vi "log analysis_gps.vi"() -> ()   [LabVIEW 2019] (continued)
02000000,d426,15824;SOL_COMPUTED,L1_FLOAT,-1.000000000,81.985870361,-51.294281006,0.0,269.498687744,180.000000000,\"631T\",17,8,8,8,04,00,20,23*d2afce59\n\tsystem status\tnormal 2 27.900000 0 0\trobot status\t132.527983\t124.834671\t7.872000\t-0.704959\t-0.765344\t1.089934\t0.295000\t0.023000\n\t\n15:13:21.0\tlog_raw\tgps_raw\t#DUALANTENNAHEADINGA,USB3,0,49.5,FINESTEERING,2107,281619.000,02000000,d426,15824;SOL_COMPUTED,L1_FLOAT,-1.000000000,81.329711914,-49.084411621,0.0,261.078948975,180.000000000,\"631T\",18,8,8,8,04,00,20,23*0738c36d\n\tsystem status\tnormal 2 28.000000 0 0\trobot status\t132.671677\t124.829898\t7.873300\t-0.689398\t-0.745768\t1.834140\t0.257000\t0.090000\n\t\n15:13:21.5\tlog_raw\tgps_raw\t#DUALANTENNAHEADINGA,USB3,0,48.0,FINESTEERING,2107,281619.500,02000000,d426,15824;SOL_COMPUTED,NARROW_FLOAT,-1.000000000,83.428977966,-43.865173340,0.0,179.560241699,180.000000000,\"631T\",20,9,9,8,04,00,20,23*fb7ce078\n\tsystem status\tnormal 2 28.000000 0 0\trobot status\t132.812972\t124.826160\t7.871700\t-0.774766\t-0.698025\t2.416964\t0.284000\t0.023000\n\t\n15:13:22.0\tlog_raw\tgps_raw\t#DUALANTENNAHEADINGA,USB3,0,48.0,FINESTEERING,2107,281620.000,02000000,d426,15824;SOL_COMPUTED,NARROW_FLOAT,-1.000000000,83.177322388,-43.462402344,0.0,179.866409302,180.000000000,\"631T\",19,9,9,8,04,00,20,23*b83e1f1b\n\tsystem status\tnormal 2 28.100000 0 0\trobot status\t132.957208\t124.822783\t7.869900\t-0.755381\t-0.663432\t2.788208\t0.242000\t0.092000\n\t\n15:13:22.5\tlog_raw\tgps_raw\t#DUALANTENNAHEADINGA,USB3,0,44.5,FINESTEERING,2107,281620.500,02000000,d426,15824;SOL_COMPUTED,NARROW_FLOAT,-1.000000000,82.434860229,-53.334503174,0.0,202.841445923,166.629974365,\"631T\",18,8,8,8,04,00,20,23*e81d707d\n\tsystem status\tnormal 2 28.100000 0 0\trobot status\t133.098233\t124.820634\t7.869100\t-0.796184\t-0.528559\t3.164091\t0.414000\t-0.170000\n\t\n15:13:23.0\tlog_raw\tgps_raw\t#INSPVAXA,USB3,0,44.5,FINESTEERING,2107,281621.000,02000000,471d,15824;INS_ALIGNMENT_COMPLETE,INS_RTKFIXED,37.37125484776,126.72233928465,7.8682,22.3000,-0.0140,0.2874,-0.0021,-0.631288099,-0.470123008,86.597817260,0.4108,0.2750,0.5022,0.1095,0.0896,0.0746,0.1671,0.1681,5.1116,0f000001,0*0301d2b2\n\tsystem status\tnormal 2 28.100000 0 0\trobot status\t133.237761\t124.817911\t7.868200\t-0.631288\t-0.470123\t3.402183\t0.271000\t0.044000\n\t\n15:13:23.5\tlog_raw\tgps_raw\t#DUALANTENNAHEADINGA,USB3,0,47.5,FINESTEERING,2107,281621.500,02000000,d426,15824;SOL_COMPUTED,L1_FLOAT,-1.000000000,79.118186951,-47.831787109,0.0,285.028137207,180.000000000,\"631T\",21,8,8,8,04,00,20,23*eceb4aca\n\tsystem status\tnormal 2 28.100000 0 0\trobot status\t133.381909\t124.815038\t7.870000\t-0.413841\t-0.414727\t3.443892\t0.363000\t-0.086000\n\t\n15:13:24.0\tlog_raw\tgps_raw\t#DUALANTENNAHEADINGA,USB3,0,47.5,FINESTEERING,2107,281622.000,02000000,d426,15824;SOL_COMPUTED,L1_FLOAT,-1.000000000,79.215469360,-46.676361084,0.0,278.801727295,180.000000000,\"631T\",21,8,8,8,04,00,20,23*2f0de768\n\tsystem status\tnormal 2 28.200000 0 0\trobot status\t133.527421\t124.811541\t7.872000\t-0.238819\t-0.445818\t3.404348\t0.278000\t0.029000\n\t\n15:13:24.5\tlog_raw\tgps_raw\t#DUALANTENNAHEADINGA,USB3,0,50.0,FINESTEERING,2107,281622.500,02008000,d426,15824;SOL_COMPUTED,NARROW_FLOAT,-1.000000000,81.357048035,-52.184570313,0.0,156.938522339,171.573028564,\"631T\",22,8,8,8,04,00,20,23*a9a2e0bd\n\tsystem status\tnormal 2 28.200000 0 0\trobot status\t133.669990\t124.807065\t7.875800\t-0.115847\t-0.480549\t3.296523\t0.293000\t0.009000\n\t\n15:13:25.0\tlog_raw\tgps_raw\t#DUALANTENNAHEADINGA,USB3,0,50.0,FINESTEERING,2107,281623.000,02008000,d426,15824;SOL_COMPUTED,NARROW_FLOAT,-1.000000000,80.926651001,-50.941162109,0.0,157.099182129,180.000000000,\"631T\",22,8,8,8,04,00,20,23*29ef00a4\n\tsystem status\tnormal 2 28.200000 0 0\trobot status\t133.812784\t124.801470\t7.879500\t0.034583\t-0.554227\t3.198241\t0.295000\t-0.009000\n\t\n15:13:25.5\tlog_raw\tgps_raw\t#DUALANTENNAHEADINGA,USB3,0,47.0,FINESTEERING,2107,281623.500,02008000,d426,15824;SOL_COMPUTED,NARROW_FLOAT,-1.000000000,74.372909546,-36.647766113,0.0,211.228378296,180.000000000,\"631T\",21,9,9,8,04,00,20,23*0d510ff3\n\tsystem status\tnormal 2 28.200000 0 0\trobot status\t133.959682\t124.793507\t7.883200\t0.412890\t-0.814601\t3.103692\t0.299000\t-0.011000\n\t\n15:13:26.0\tlog_raw\tgps_raw\t#DUALANTENNAHEADINGA,USB3,0,47.0,FINESTEERING,2107,281624.000,02008000,d426,15824;SOL_COMPUTED,NARROW_FLOAT,-1.000000000,74.676368713,-33.559204102,0.0,205.690567017,180.000000000,\"631T\",20,9,9,8,04,00,20,23*f648ddb8\n\tsystem status\tnormal 2 28.200000 0 0\trobot status\t134.101094\t124.785415\t7.887300\t0.610602\t-0.952915\t3.005464\t0.297000\t-0.013000\n\t\n15:13:26.5\tlog_raw\tgps_raw\t#DUALANTENNAHEADINGA,USB3,0,47.5,FINESTEERING,2107,281624.500,02008000,d426,15824;SOL_COMPUTED,NARROW_FLOAT,-1.000000000,78.385162354,-52.385925293,0.0,193.963928223,180.000000000,\"631T\",19,8,8,8,04,00,20,23*14d467ea\n\tsystem status\tnormal 2 28.200000 0 0\trobot status\t134.242225\t124.778426\t7.889200\t0.752717\t-1.000787\t2.886940\t0.295000\t-0.016000\n\t\n15:13:27.0\tlog_raw\tgps_raw\t#DUALANTENNAHEADINGA,USB3,0,47.5,FINESTEERING,2107,281625.000,02008000,d426,15824;SOL_COMPUTED,NARROW_FLOAT,-1.000000000,78.697448730,-55.840881348,0.0,201.517425537,180.000000000,\"631T\",20,8,8,8,04,00,20,23*2125c3e9\n\tsystem status\tnormal 2 28.200000 0 0\trobot status\t134.384632\t124.770462\t7.890500\t0.886447\t-0.920314\t2.761621\t0.298000\t-0.007000\n\t\n15:13:27.5\tlog_raw\tgps_raw\t#DUALANTENNAHEADINGA,USB3,0,50.0,FINESTEERING,2107,281625.500,02008000,d426,15824;SOL_COMPUTED,NARROW_FLOAT,-1.000000000,76.255996704,-44.440551758,0.0,192.652679443,180.000000000,\"631T\",21,8,8,8,04,00,20,23*2ef6fdf0\n\tsystem status\tnormal 2 28.200000 0 0\trobot status\t134.527815\t124.762984\t7.891800\t1.028451\t-0.676309\t2.638165\t0.297000\t-0.013000\n\t\n15:13:28.0\tlog_raw\tgps_raw\t#DUALANTENNAHEADINGA,USB3,0,50.0,FINESTEERING,2107,281626.000,02008000,d426,15824;SOL_COMPUTED,NARROW_FLOAT,-1.000000000,76.051048279,-42.751831055,0.0,190.193801880,180.000000000,\"631T\",19,8,8,8,04,00,20,23*71df93c1\n\tsystem status\tnormal 2 28.200000 0 0\trobot status\t134.672251\t124.753527\t7.893800\t1.313181\t-0.400313\t2.489606\t0.294000\t-0.014000\n\t\n15:13:28.5\tlog_raw\tgps_raw\t\tsystem status\tnormal 2 28.200000 0 0\trobot status\t134.821411\t124.744984\t7.894300\t1.448971\t-0.286102\t2.371589\t0.296000\t-0.007000\n\t\n15:13:29.0\tlog_raw\tgps_raw\t#DUALANTENNAHEADINGA,USB3,0,49.0,FINESTEERING,2107,281627.000,02000000,d426,15824;SOL_COMPUTED,NARROW_FLOAT,-1.000000000,74.827011108,-47.434204102,0.0,215.584564209,180.000000000,\"631T\",20,6,6,6,04,00,20,03*11cc19a9\n\tsystem status\tnormal 2 28.200000 0 0\trobot status\t134.968968\t124.735417\t7.895300\t1.459946\t-0.353992\t2.207850\t0.302000\t-0.011000\n\t\n15:13:29.5\tlog_raw\tgps_raw\t#DUALANTENNAHEADINGA,USB3,0,50.0,FINESTEERING,2107,281627.500,02000000,d426,15824;SOL_COMPUTED,NARROW_FLOAT,-1.000000000,76.736885071,-60.461914063,0.0,257.944244385,180.000000000,\"631T\",20,6,6,6,04,00,20,03*64121f5a\n\tsystem status\tnormal 2 28.200000 0 0\trobot status\t135.110611\t124.726484\t7.897200\t1.391975\t-0.391573\t2.021625\t0.300000\t-0.012000\n\t\n15:13:30.0\tlog_raw\tgps_raw\t#DUALANTENNAHEADINGA,USB3,0,50.0,FINESTEERING,2107,281628.000,02000000,d426,15824;SOL_COMPUTED,NARROW_FLOAT,-1.000000000,76.336128235,-57.847045898,0.0,256.018859863,180.000000000,\"631T\",20,6,6,6,04,00,20,03*cae9a6c4\n\tsystem status\tnormal 2 28.200000 0 0\trobot status\t135.258314\t124.716625\t7.899300\t1.303987\t-0.581408\t1.863464\t0.296000\t-0.010000\n\t\n15:13:30.5\tlog_raw\tgps_raw\t#DUALANTENNAHEADINGA,USB3,0,49.0,FINESTEERING,2107,281628.500,02000000,d426,15824;SOL_COMPUTED,NARROW_FLOAT,-1.000000000,75.922164917,-51.811248779,0.0,196.475540161,180.000000000,\"631T\",21,6,6,6,04,00,20,03*71a30e30\n\tsystem status\tnormal 2 28.200000 0 0\trobot status\t135.405242\t124.709408\t7.900300\t1.225879\t-0.705011\t1.692036\t0.301000\t-0.006000\n\t\n15:13:31.0\tlog_raw\tgps_raw\t#DUALANTENNAHEADINGA,USB3,0,49.0,FINESTEERING,2107,281629.000,02000000,d426,15824;SOL_COMPUTED,NARROW_FLOAT,-1.000000000,75.688812256,-51.816131592,0.0,200.071166992,180.000000000,\"631T\",21,6,6,6,04,00,20,03*05442491\n\tsystem status\tnormal 2 28.200000 0 0\trobot status\t135.549471\t124.701412\t7.901000\t1.137564\t-0.721640\t1.522246\t0.302000\t-0.011000\n\t\n15:13:31.5\tlog_raw\tgps_raw\t#DUALANTENNAHEADINGA,USB3,0,47.0,FINESTEERING,2107,281629.500,02000000,d426,15824;SOL_COMPUTED,NARROW_FLOAT,-1.000000000,76.706954956,-45.822814941,0.0,158.336380005,180.000000000,\"631T\",21,7,7,6,04,00,20,03*a7b53285\n\tsystem status\tnormal 2 28.200000 0 0\trobot status\t135.689730\t124.694593\t7.901700\t1.081795\t-0.675095\t1.331584\t0.298000\t-0.003000\n\t\n15:13:32.0\tlog_raw\tgps_raw\t#DUALANTENNAHEADINGA,USB3,0,47.0,FINESTEERING,2107,281630.000,02000000,d426,15824;SOL_COMPUTED,NARROW_FLOAT,-1.000000000,76.392150879,-45.545715332,0.0,160.233947754,180.000000000,\"631T\",20,7,7,6,04,00,20,03*a337a603\n\tsystem status\tnormal 2 28.200000 0 0\trobot status\t135.832695\t124.687325\t7.902200\t0.907226\t-0.591803\t1.171661\t0.292000\t0.000000\n\t\n15:13:32.5\tlog_raw\tgps_raw\t#DUALANTENNAHEADINGA,USB3,0,50.0,FINESTEERING,2107,281630.500,02000000,d426,15824;SOL_COMPUTED,NARROW_FLOAT,-1.000000000,73.576385498,-34.237976074,0.0,224.892852783,180.000000000,\"631T\",20,7,7,6,04,00,20,03*509d4fa7\n\tsystem status\tnormal 2 28.200000 0 0\trobot status\t135.975938\t124.680414\t7.903900\t0.750666\t-0.654550\t1.015174\t0.302000\t-0.002000\n\t\n15:13:33.0\tlog_raw\tgps_raw\t#DUALANTENNAHEADINGA,USB3,0,50.0,FINESTEERING,2107,281631.000,02000000,d426,15824;SOL_COMPUTED,NARROW_FLOAT,-1.000000000,73.801551819,-34.781646729,0.0,227.056274414,180.000000000,\"631T\",20,7,7,6,04,00,20,03*62a89227\n\tsystem status\tnormal 2 28.200000 0 0\trobot status\t136.111228\t124.672284\t7.907100\t0.620165\t-0.528572\t0.833307\t0.298000\t0.000000\n\t\n15:13:33.5\tlog_raw\tgps_raw\t#DUALANTENNAHEADINGA,USB3,0,48.5,FINESTEERING,2107,281631.500,02000000,d426,15824;SOL_COMPUTED,NARROW_FLOAT,-1.000000000,72.331886292,-39.270935059,0.0,208.219329834,180.000000000,\"631T\",20,6,6,6,04,00,20,03*b4f25b02\n\tsystem status\tnormal 2 28.200000 0 0\trobot status\t136.251123\t124.665216\t7.908000\t0.625068\t-0.387180\t0.705750\t0.296000\t0.006000\n\t\n15:13:34.0\tlog_raw\tgps_raw\t#DUALANTENNAHEADINGA,USB3,0,48.5,FINESTEERING,2107,281632.000,02000000,d426,15824;SOL_COMPUTED,NARROW_FLOAT,-1.000000000,72.392997742,-44.277435303,0.0,216.308242798,180.000000000,\"631T\",20,6,6,6,04,00,20,03*f92d3de0\n\tsystem status\tnormal 2 28.200000 0 0\trobot status\t136.388999\t124.657518\t7.909100\t0.522944\t-0.320117\t0.535098\t0.295000\t-0.005000\n\t\n15:13:34.5\tlog_raw\tgps_raw\t#DUALANTENNAHEADINGA,USB3,0,50.5,FINESTEERING,2107,281632.500,02000000,d426,15824;SOL_COMPUTED,NARROW_FLOAT,-1.000000000,70.524742126,-43.222106934,0.0,187.663330078,180.000000000,\"631T\",20,6,6,6,04,00,20,03*23e53db0\n\tsystem status\tnormal 2 28.200000 0 0\trobot status\t136.527493\t124.649932\t7.910000\t0.480007\t-0.230660\t0.402714\t0.302000\t-0.002000\n\t\n15:13:35.0\tlog_raw\tgps_raw\t\tsystem status\tnormal 2 28.200000 0 0\trobot status\t136.664747\t124.641530\t7.912700\t0.383209\t-0.068987\t0.273789\t0.299000\t0.000000\n\t\n15:13:35.5\tlog_raw\tgps_raw\t\tsystem status\tnormal 2 28.200000 0 0\trobot status\t136.804079\t124.633410\t7.915200\t0.323321\t0.031538\t0.175839\t0.295000\t0.000000\n\t\n15:13:36.0\tlog_raw\tgps_raw\t\tsystem status\tnormal 2 28.200000 0 0\trobot status\t136.946767\t124.624659\t7.917300\t0.214120\t0.032979\t0.078057\t0.301000\t0.004000\n\t\n15:13:36.5\tlog_raw\tgps_raw\t#DUALANTENNAHEADINGA,USB3,0,49.5,FINESTEERING,2107,281634.500,02000000,d426,15824;SOL_COMPUTED,NARROW_FLOAT,-1.000000000,74.599754333,-34.968170166,0.0,186.703521729,180.000000000,\"631T\",21,8,8,8,04,00,20,33*c6f47f17\n\tsystem status\tnormal 2 28.200000 0 0\trobot status\t137.089583\t124.616962\t7.919700\t0.037424\t-0.007948\t-0.020745\t0.304000\t0.008000\n\t\n15:13:37.0\tlog_raw\tgps_raw\t#DUALANTENNAHEADINGA,USB3,0,49.5,FINESTEERING,2107,281635.000,02000000,d426,15824;SOL_COMPUTED,NARROW_FLOAT,-1.000000000,74.584259033,-34.924865723,0.0,186.240829468,180.000000000,\"631T\",21,8,8,8,04,00,20,33*9c697b75\n\tsystem status\tnormal 2 28.200000 0 0\trobot status\t137.230387\t124.607716\t7.921700\t-0.027327\t-0.162985\t-0.124730\t0.299000\t0.008000\n\t\n15:13:37.5\tlog_raw\tgps_raw\t#DUALANTENNAHEADINGA,USB3,0,46.5,FINESTEERING,2107,281635.500,02000000,d426,15824;SOL_COMPUTED,NARROW_FLOAT,-1.000000000,67.143241882,-41.090057373,0.0,270.678344727,180.000000000,\"631T\",21,8,8,8,04,00,20,23*92e43030\n\tsystem status\tnormal 2 28.200000 0 0\trobot status\t137.372263\t124.599397\t7.922900\t-0.076547\t-0.321066\t-0.217362\t0.301000\t0.007000\n\t\n15:13:38.0\tlog_raw\tgps_raw\t#INSPVAXA,USB3,0,46.5,FINESTEERING,2107,281636.050,02000000,471d,15824;INS_ALIGNMENT_COMPLETE,INS_RTKFIXED,37.37125277821,126.72238773089,7.9249,22.3000,-0.0472,0.2751,0.0261,0.033461112,-0.337994912,90.276833598,0.4107,0.2743,0.5040,0.1102,0.0902,0.0747,0.1666,0.1669,5.1095,0f000001,0*fb0d7dd5\n\tsystem status\tnormal 2 28.200000 0 0\trobot status\t137.529050\t124.588153\t7.924900\t0.033461\t-0.337995\t-0.276834\t0.298000\t0.005000\n\t\n15:13:38.5\tlog_raw\tgps_raw\t#INSPVAXA,USB3,0,49.0,FINESTEERING,2107,281636.550,02000000,471d,15824;INS_ALIGNMENT_COMPLETE,INS_RTKFIXED,37.37125270683,126.72238933988,7.9258,22.3000,-0.0404,0.2826,0.0202,-0.092396581,-0.312496368,90.344441421,0.4107,0.2743,0.5040,0.1102,0.0902,0.0747,0.1666,0.1669,5.1095,0f000001,0*2ea03c91\n\tsystem status\tnormal 2 28.200000 0 0\trobot status\t137.671572\t124.580228\t7.925800\t-0.092397\t-0.312496\t-0.344441\t0.304000\t0.006000\n\t\n15:13:39.0\tlog_raw\tgps_raw\t\tsystem status\tnormal 2 28.200000 0 0\trobot status\t137.796732\t124.571946\t7.926200\t-0.126269\t-0.143738\t-0.384547\t0.296000\t0.008000\n\t\n15:13:39.5\tlog_raw\tgps_raw\t\tsystem status\tnormal 2 28.200000 0 0\trobot status\t137.940609\t124.562478\t7.926700\t-0.091947\t-0.054945\t-0.381561\t0.244000\t0.066000\n\t\n15:13:40.0\tlog_raw\tgps_raw\t#DUALANTENNAHEADINGA,USB3,0,45.5,FINESTEERING,2107,281638.000,02000000,d426,15824;SOL_COMPUTED,L1_FLOAT,-1.000000000,68.590065002,-38.051055908,0.0,183.932281494,180.000000000,\"631T\",19,6,6,6,04,00,20,03*7caf4eb9\n\tsystem status\tnormal 2 28.200000 0 0\trobot status\t138.081185\t124.552915\t7.928500\t-0.095749\t-0.090492\t-0.295128\t0.301000\t0.006000\n\t\n15:13:40.5\tlog_raw\tgps_raw\t#DUALANTENNAHEADINGA,USB3,0,46.5,FINESTEERING,2107,281638.500,02000000,d426,15824;SOL_COMPUTED,NARROW_FLOAT,-1.000000000,65.883399963,-37.877685547,0.0,260.404785156,180.000000000,\"631T\",19,6,6,6,04,00,20,03*2dc9451b\n\tsystem status\tnormal 2 28.200000 0 0\trobot status\t138.222022\t124.543481\t7.929100\t-0.131894\t-0.163924\t-0.209489\t0.369000\t-0.101000\n\t\n15:13:41.0\tlog_raw\tgps_raw\t#DUALANTENNAHEADINGA,USB3,0,46.5,FINESTEERING,2107,281639.000,02000000,d426,15824;SOL_COMPUTED,NARROW_FLOAT,-1.000000000,66.000267029,-38.685607910,0.0,260.610321045,180.000000000,\"631T\",20,6,6,6,04,00,20,03*4d0efe6f\n\tsystem status\tnormal 2 28.200000 0 0\trobot status\t138.363859\t124.533398\t7.929800\t-0.101029\t-0.169552\t-0.100452\t0.253000\t0.068000\n\t\n15:13:41.5\tlog_raw\tgps_raw\t#DUALANTENNAHEADINGA,USB3,0,48.5,FINESTEERING,2107,281639.500,02000000,d426,15824;SOL_COMPUTED,L1_FLOAT,-1.000000000,75.249496460,-42.510375977,0.0,208.045684814,180.000000000,\"631T\",21,6,6,6,04,00,20,03*5f68b654\n\tsystem status\tnormal 2 28.100000 0 0\trobot status\t138.507917\t124.525404\t7.930000\t-0.080780\t-0.161525\t0.054370\t0.379000\t-0.118000\n\t\n15:13:42.0\tlog_raw\tgps_raw\t#INSPVAXA,USB3,0,48.5,FINESTEERING,2107,281640.050,02000000,471d,15824;INS_ALIGNMENT_COMPLETE,INS_RTKFIXED,37.37125214763,126.72240056337,7.9297,22.3000,-0.0135,0.2579,0.0068,-0.286062471,-0.323666659,89.847152280,0.4125,0.2764,0.5060,0.1103,0.0900,0.0751,0.1666,0.1668,5.0988,0f000001,0*ba23ac07\n\tsystem status\tnormal 2 28.100000 0 0\trobot status\t138.665730\t124.518149\t7.929700\t-0.286062\t-0.323667\t0.152848\t0.293000\t0.019000\n\t\n15:13:42.5\tlog_raw\tgps_raw\t#INSPVAXA,USB3,0,48.0,FINESTEERING,2107,281640.550,02000000,471d,15824;INS_ALIGNMENT_COMPLETE,INS_RTKFIXED,37.37125209177,126.72240219164,7.9302,22.3000,-0.0088,0.2910,0.0070,-0.402825577,-0.342049421,89.793656004,0.4125,0.2764,0.5060,0.1103,0.0900,0.0751,0.1666,0.1668,5.0988,0f000001,0*83e377ec\n\tsystem status\tnormal 2 28.100000 0 0\trobot status\t138.809960\t124.511947\t7.930200\t-0.402826\t-0.342049\t0.206344\t0.297000\t0.007000\n\t\n15:13:43.0\tlog_raw\tgps_raw\t\tsystem status\tnormal 2 28.100000 0 0\trobot status\t138.938093\t124.505250\t7.930200\t-0.365984\t-0.316955\t0.417263\t0.357000\t-0.091000\n\t\n15:13:43.5\tlog_raw\tgps_raw\t\tsystem status\tnormal 2 28.100000 0 0\trobot status\t139.083168\t124.498292\t7.930000\t-0.534292\t-0.438853\t0.507811\t0.211000\t0.110000\n\t\n15:13:44.0\tlog_raw\tgps_raw\t\tsystem status\tnormal 2 28.100000 0 0\trobot status\t139.226269\t124.491404\t7.929600\t-0.722782\t-0.398658\t0.533081\t0.406000\t-0.162000\n\t\n15:13:44.5\tlog_raw\tgps_raw\t\tsystem status\tnormal 2 28.200000 0 0\trobot status\t139.369835\t124.484513\t7.927700\t-0.695260\t-0.251085\t0.563271\t0.261000\t0.043000\n\t\n15:13:45.0\tlog_raw\tgps_raw\t#INSPVAXA,USB3,0,49.5,FINESTEERING,2107,281643.050,02000000,471d,15824;INS_ALIGNMENT_COMPLETE,INS_RTKFIXED,37.37125177239,126.72241029930,7.9253,22.3000,-0.0184,0.2626,0.0057,-0.672263501,-0.094085877,89.482974840,0.4115,0.2769,0.5079,0.1098,0.0898,0.0750,0.1665,0.1668,5.0987,0f000001,0*08f45476\n\tsystem status\tnormal 2 28.100000 0 0\trobot status\t139.528123\t124.476489\t7.925300\t-0.672264\t-0.094086\t0.517025\t0.352000\t-0.107000\n\t\n15:13:45.5\tlog_raw\tgps_raw\t\tsystem status\tnormal 2 28.200000 0 0\trobot status\t139.657963\t124.469457\t7.924200\t-0.620368\t-0.040100\t0.509446\t0.290000\t0.006000\n\t\n15:13:46.0\tlog_raw\tgps_raw\t#INSPVAXA,USB3,0,45.0,FINESTEERING,2107,281644.050,02000000,471d,15824;INS_ALIGNMENT_COMPLETE,INS_RTKFIXED,37.37125163862,126.72241353138,7.9238,22.3000,-0.0195,0.2934,0.0047,-0.764058138,0.046945351,89.556014373,0.4117,0.2771,0.5083,0.1098,0.0898,0.0750,0.1665,0.1667,5.0999,0f000001,0*ca60484a\n\tsystem status\tnormal 2 28.200000 0 0\trobot status\t139.814415\t124.461638\t7.923800\t-0.764058\t0.046945\t0.443986\t0.313000\t-0.019000\n\t\n15:13:46.5\tlog_raw\tgps_raw\t#INSPVAXA,USB3,0,49.0,FINESTEERING,2107,281644.550,02000000,471d,15824;INS_ALIGNMENT_COMPLETE,INS_RTKFIXED,37.37125159291,126.72241516710,7.9252,22.3000,-0.0125,0.2656,0.0050,-0.825704601,0.105733929,89.608837523,0.4117,0.2771,0.5083,0.1098,0.0898,0.0750,0.1665,0.1667,5.0999,0f000001,0*afd891ca\n\tsystem status\tnormal 2 28.200000 0 0\trobot status\t139.959304\t124.456563\t7.925200\t-0.825705\t0.105734\t0.391162\t0.286000\t-0.009000\n\t\n15:13:47.0\tlog_raw\tgps_raw\t#INSPVAXA,USB3,0,49.0,FINESTEERING,2107,281645.050,02000000,471d,15824;INS_ALIGNMENT_COMPLETE,INS_RTKFIXED,37.37125153841,126.72241684941,7.9264,22.3000,-0.0138,0.2766,0.0005,-0.782015483,0.115845462,89.701566718,0.4112,0.2772,0.5084,0.1097,0.0898,0.0750,0.1665,0.1667,5.1015,0f000001,0*e301f266\n\tsystem status\tnormal 2 28.200000 0 0\trobot status\t140.108321\t124.450511\t7.926400\t-0.782015\t0.115845\t0.298433\t0.294000\t-0.003000\n\t\n15:13:47.5\tlog_raw\tgps_raw\t\tsystem status\tnormal 2 28.200000 0 0\trobot status\t140.237450\t124.444010\t7.925800\t-0.680854\t-0.008764\t0.272391\t0.302000\t-0.013000\n\t\n15:13:48.0\tlog_raw\tgps_raw\t#INSPVAXA,USB3,0,51.0,FINESTEERING,2107,281646.050,02000000,471d,15824;INS_ALIGNMENT_COMPLETE,INS_RTKFIXED,37.37125141044,126.72242010916,7.9241,22.3000,-0.0145,0.2894,0.0046,-0.683948152,-0.106427214,89.829684662,0.4110,0.2773,0.5083,0.1096,0.0899,0.0750,0.1665,0.1667,5.1032,0f000001,0*7e3f8e98\n\tsystem status\tnormal 2 28.200000 0 0\trobot status\t140.397064\t124.436304\t7.924100\t-0.683948\t-0.106427\t0.170315\t0.295000\t-0.013000\n\t\n15:13:48.5\tlog_raw\tgps_raw\t\tsystem status\tnormal 2 28.200000 0 0\trobot status\t140.529109\t124.428553\t7.922100\t-0.559415\t-0.144844\t0.061968\t0.288000\t-0.017000\n\t\n15:13:49.0\tlog_raw\tgps_raw\t\tsystem status\tnormal 2 28.200000 0 0\trobot status\t140.670749\t124.420683\t7.920600\t-0.646021\t-0.153969\t-0.024187\t0.298000\t-0.013000\n\t\n15:13:49.5\tlog_raw\tgps_raw\t\tsystem status\tnormal 2 28.200000 0 0\trobot status\t140.810969\t124.412523\t7.920300\t-0.671934\t0.006720\t-0.060655\t0.301000\t-0.013000\n\t\n15:13:50.0\tlog_raw\tgps_raw\t\tsystem status\tnormal 2 28.200000 0 0\trobot status\t140.956641\t124.403565\t7.920000\t-0.694143\t0.279069\t-0.163248\t0.292000\t-0.017000\n\t\n15:13:50.5\tlog_raw\tgps_raw\t#INSPVAXA,USB3,0,50.5,FINESTEERING,2107,281648.550,02000000,471d,15824;INS_ALIGNMENT_COMPLETE,INS_RTKFIXED,37.37125104211,126.72242819820,7.9192,22.3000,-0.0057,0.2779,0.0043,-0.865746254,0.658403910,90.332036751,0.4101,0.2775,0.5080,0.1095,0.0899,0.0749,0.1664,0.1667,5.1060,0f000001,0*c1bd000c\n\tsystem status\tnormal 2 28.200000 0 0\trobot status\t141.113578\t124.395413\t7.919200\t-0.865746\t0.658404\t-0.332037\t0.298000\t-0.011000\n\t\n15:13:51.0\tlog_raw\tgps_raw\t#INSPVAXA,USB3,0,47.0,FINESTEERING,2107,281649.050,02000000,471d,15824;INS_ALIGNMENT_COMPLETE,INS_RTKFIXED,37.37125095950,126.72242975720,7.9195,22.3000,-0.0170,0.2957,0.0033,-0.943502690,0.808287959,90.436788993,0.4102,0.2776,0.5078,0.1095,0.0899,0.0749,0.1664,0.1667,5.1072,0f000001,0*5974bd17\n\tsystem status\tnormal 2 28.200000 0 0\trobot status\t141.251672\t124.386242\t7.919500\t-0.943503\t0.808288\t-0.436789\t0.297000\t-0.013000\n\t\n15:13:51.5\tlog_raw\tgps_raw\t#INSPVAXA,USB3,0,47.0,FINESTEERING,2107,281649.550,02000000,471d,15824;INS_ALIGNMENT_COMPLETE,INS_RTKFIXED,37.37125085766,126.72243133912,7.9203,22.3000,-0.0165,0.2929,0.0110,-0.815482674,0.895195605,90.550000781,0.4102,0.2776,0.5078,0.1095,0.0899,0.0749,0.1664,0.1667,5.1072,0f000001,0*975e6869\n\tsystem status\tnormal 2 28.200000 0 0\trobot status\t141.391796\t124.374937\t7.920300\t-0.815483\t0.895196\t-0.550001\t0.294000\t-0.017000\n\t\n15:13:52.0\tlog_raw\tgps_raw\t#INSPVAXA,USB3,0,47.0,FINESTEERING,2107,281650.050,02000000,471d,15824;INS_ALIGNMENT_COMPLETE,INS_RTKFIXED,37.37125074410,126.72243299345,7.9208,22.3000,-0.0194,0.2944,0.0151,-0.654661826,0.805584356,90.730688305,0.4111,0.2776,0.5078,0.1096,0.0901,0.0749,0.1664,0.1667,5.1084,0f000001,0*7ee54a6b\n\tsystem status\tnormal 2 28.200000 0 0\trobot status\t141.538333\t124.362331\t7.920800\t-0.654662\t0.805584\t-0.730688\t0.292000\t-0.013000\n\t\n15:13:52.5\tlog_raw\tgps_raw\t#INSPVAXA,USB3,0,49.5,FINESTEERING,2107,281650.550,02000000,471d,15824;INS_ALIGNMENT_COMPLETE,INS_RTKFIXED,37.37125062801,126.72243464345,7.9218,22.3000,-0.0206,0.2968,0.0101,-0.581641852,0.404768185,90.963959440,0.4111,0.2776,0.5078,0.1096,0.0901,0.0749,0.1664,0.1667,5.1084,0f000001,0*f2a4c14e\n\tsystem status\tnormal 2 28.200000 0 0\trobot status\t141.684488\t124.349444\t7.921800\t-0.581642\t0.404768\t-0.963959\t0.299000\t-0.009000\n\t\n15:13:53.0\tlog_raw\tgps_raw\t#INSPVAXA,USB3,0,49.5,FINESTEERING,2107,281651.050,02000000,471d,15824;INS_ALIGNMENT_COMPLETE,INS_RTKFIXED,37.37125051285,126.72243625014,7.9235,22.3000,-0.0268,0.3045,0.0175,-0.662592503,0.202583400,91.123013334,0.4115,0.2778,0.5076,0.1098,0.0901,0.0749,0.1663,0.1667,5.1090,0f000001,0*216f234f\n\tsystem status\tnormal 2 28.200000 0 0\trobot status\t141.826806\t124.336661\t7.923500\t-0.662593\t0.202583\t-1.123013\t0.302000\t-0.010000\n\t\n15:13:53.5\tlog_raw\tgps_raw\t\tsystem status\tnormal 2 28.200000 0 0\trobot status\t141.956980\t124.325325\t7.923600\t-0.638179\t0.078223\t-1.263436\t0.295000\t-0.003000\n\t\n15:13:54.0\tlog_raw\tgps_raw\t#INSPVAXA,USB3,0,45.5,FINESTEERING,2107,281652.050,02000000,471d,15824;INS_ALIGNMENT_COMPLETE,INS_RTKFIXED,37.37125028624,126.72243951930,7.9245,22.3000,-0.0369,0.2898,0.0166,-0.721183306,0.056680654,91.387520198,0.4416,0.2813,0.5208,0.1150,0.0908,0.0760,0.1664,0.1673,5.1091,0f000001,0*25228c2c\n\tsystem status\tnormal 2 28.200000 0 0\trobot status\t142.116382\t124.311506\t7.924500\t-0.721183\t0.056681\t-1.387520\t0.304000\t-0.005000\n\t\n15:13:54.5\tlog_raw\tgps_raw\t\tsystem status\tnormal 2 28.200000 0 0\trobot status\t142.244213\t124.299152\t7.925200\t-0.610039\t0.089492\t-1.534593\t0.296000\t-0.010000\n\t\n15:13:55.0\tlog_raw\tgps_raw\t#INSPVAXA,USB3,0,47.5,FINESTEERING,2107,281653.050,02000000,471d,15824;INS_ALIGNMENT_COMPLETE,INS_RTKFIXED,37.37125003154,126.72244272682,7.9262,22.3000,-0.0470,0.2934,0.0145,-0.464349418,0.202545011,91.639204054,0.4699,0.2842,0.5361,0.1187,0.0913,0.0769,0.1664,0.1677,5.1090,0f000001,0*2b109b71\n\tsystem status\tnormal 2 28.200000 0 0\trobot status\t142.400499\t124.283233\t7.926200\t-0.464349\t0.202545\t-1.639204\t0.302000\t0.000000\n\t\n15:13:55.5\tlog_raw\tgps_raw\t#INSPVAXA,USB3,0,47.5,FINESTEERING,2107,281653.550,02000000,471d,15824;INS_ALIGNMENT_COMPLETE,INS_RTKFIXED,37.37124990486,126.72244436292,7.9283,22.3000,-0.0470,0.2912,0.0231,-0.374405811,0.178417245,91.756627389,0.4699,0.2842,0.5361,0.1187,0.0913,0.0769,0.1664,0.1677,5.1090,0f000001,0*1daf5624\n\tsystem status\tnormal 2 28.200000 0 0\trobot status\t142.545422\t124.269171\t7.928300\t-0.374406\t0.178417\t-1.756627\t0.304000\t-0.001000\n\t\n15:13:56.0\tlog_raw\tgps_raw\t#INSPVAXA,USB3,0,47.5,FINESTEERING,2107,281654.050,02000000,471d,15824;INS_ALIGNMENT_COMPLETE,INS_RTKFIXED,37.37124978665,126.72244599017,7.9303,22.3000,-0.0443,0.2911,0.0221,-0.533917833,0.012272263,91.868776619,0.4905,0.2861,0.5500,0.1206,0.0913,0.0777,0.1663,0.1679,5.1083,0f000001,0*b5797700\n\tsystem status\tnormal 2 28.200000 0 0\trobot status\t142.689562\t124.256049\t7.930300\t-0.533918\t0.012272\t-1.868777\t0.303000\t0.003000\n\t\n15:13:56.5\tlog_raw\tgps_raw\t#INSPVAXA,USB3,0,50.0,FINESTEERING,2107,281654.550,02000000,471d,15824;INS_ALIGNMENT_COMPLETE,INS_RTKFIXED,37.37124968143,126.72244761542,7.9319,22.3000,-0.0412,0.3115,0.0211,-0.670904223,-0.153080533,91.963880825,0.4905,0.2861,0.5500,0.1206,0.0913,0.0777,0.1663,0.1679,5.1083,0f000001,0*92b26d05\n\tsystem status\tnormal 2 28.200000 0 0\trobot status\t142.833524\t124.244369\t7.931900\t-0.670904\t-0.153081\t-1.963881\t0.302000\t0.006000\n\t\n15:13:57.0\tlog_raw\tgps_raw\t#INSPVAXA,USB3,0,50.0,FINESTEERING,2107,281655.050,02000000,471d,15824;INS_ALIGNMENT_COMPLETE,INS_RTKFIXED,37.37124956365,126.72244929570,7.9335,22.3000,-0.0287,0.2866,0.0163,-0.633101230,-0.384686660,92.084311938,0.4910,0.2854,0.5548,0.1194,0.0909,0.0776,0.1663,0.1676,5.1075,0f000001,0*34863e77\n\tsystem status\tnormal 2 28.200000 0 0\trobot status\t142.982360\t124.231295\t7.933500\t-0.633101\t-0.384687\t-2.084312\t0.297000\t0.000000\n\t\n15:13:57.5\tlog_raw\tgps_raw\t#INSPVAXA,USB3,0,45.0,FINESTEERING,2107,281655.550,02000000,471d,15824;INS_ALIGNMENT_COMPLETE,INS_RTKFIXED,37.37124945994,126.72245094764,7.9362,22.3000,-0.0311,0.2897,0.0132,-0.611375277,-0.501090520,92.141784733,0.4910,0.2854,0.5548,0.1194,0.0909,0.0776,0.1663,0.1676,5.1075,0f000001,0*d10d29d1\n\tsystem status\tnormal 2 28.200000 0 0\trobot status\t143.128686\t124.219782\t7.936200\t-0.611375\t-0.501091\t-2.141785\t0.299000\t0.006000\n\t\n15:13:58.0\tlog_raw\tgps_raw\t#INSPVAXA,USB3,0,45.0,FINESTEERING,2107,281656.050,02000000,471d,15824;INS_ALIGNMENT_COMPLETE,INS_RTKFIXED,37.37124935153,126.72245256975,7.9391,22.3000,-0.0386,0.2989,0.0132,-0.570389168,-0.459677112,92.213933334,0.4880,0.2845,0.5571,0.1182,0.0907,0.0775,0.1662,0.1674,5.1068,0f000001,0*a2bfb50c\n\tsystem status\tnormal 2 28.200000 0 0\trobot status\t143.272370\t124.207748\t7.939100\t-0.570389\t-0.459677\t-2.213933\t0.302000\t0.005000\n\t\n15:13:58.5\tlog_raw\tgps_raw\t\tsystem status\tnormal 2 28.200000 0 0\trobot status\t143.415453\t124.194029\t7.938500\t-0.577962\t-0.370357\t-2.256851\t0.300000\t0.004000\n\t\n15:13:59.0\tlog_raw\tgps_raw\t#INSPVAXA,USB3,0,48.5,FINESTEERING,2107,281657.050,02000000,471d,15824;INS_ALIGNMENT_COMPLETE,INS_RTKFIXED,37.37124909812,126.72245582569,7.9380,22.3000,-0.0275,0.2897,0.0035,-0.469663173,-0.125718508,92.311505672,0.4756,0.2829,0.5533,0.1158,0.0905,0.0770,0.1661,0.1672,5.1057,0f000001,0*07acf302\n\tsystem status\tnormal 2 28.200000 0 0\trobot status\t143.560776\t124.179618\t7.938000\t-0.469663\t-0.125719\t-2.311506\t0.300000\t0.006000\n\t\n15:13:59.5\tlog_raw\tgps_raw\t#INSPVAXA,USB3,0,45.5,FINESTEERING,2107,281657.550,02000000,471d,15824;INS_ALIGNMENT_COMPLETE,INS_RTKFIXED,37.37124898406,126.72245743531,7.9384,22.3000,-0.0303,0.2838,-0.0006,-0.590912103,0.021707043,92.352601821,0.4756,0.2829,0.5533,0.1158,0.0905,0.0770,0.1661,0.1672,5.1057,0f000001,0*08773687\n\tsystem status\tnormal 2 28.200000 0 0\trobot status\t143.703353\t124.166957\t7.938400\t-0.590912\t0.021707\t-2.352602\t0.283000\t0.026000\n\t\n15:14:00.0\tlog_raw\tgps_raw\t#INSPVAXA,USB3,0,45.5,FINESTEERING,2107,281658.050,02000000,471d,15824;INS_ALIGNMENT_COMPLETE,INS_RTKFIXED,37.37124887128,126.72245908204,7.9396,22.3000,-0.0216,0.3115,-0.0012,-0.683943291,-0.073848905,92.385513763,0.4705,0.2822,0.5519,0.1155,0.0906,0.0768,0.1661,0.1672,5.1055,0f000001,0*f6b19920\n\tsystem status\tnormal 2 28.200000 0 0\trobot status\t143.849218\t124.154437\t7.939600\t-0.683943\t-0.073849\t-2.385514\t0.313000\t-0.008000\n\t\n15:14:00.5\tlog_raw\tgps_raw\t#INSPVAXA,USB3,0,47.0,FINESTEERING,2107,281658.550,02000000,471d,15824;INS_ALIGNMENT_COMPLETE,INS_RTKFIXED,37.37124877139,126.72246069396,7.9391,22.3000,-0.0206,0.3045,-0.0060,-0.740293612,-0.175653816,92.281973521,0.4705,0.2822,0.5519,0.1155,0.0906,0.0768,0.1661,0.1672,5.1055,0f000001,0*bcff9c67\n\tsystem status\tnormal 2 28.100000 0 0\trobot status\t143.991999\t124.143349\t7.939100\t-0.740294\t-0.175654\t-2.281974\t0.362000\t-0.092000\n\t\n15:14:01.0\tlog_raw\tgps_raw\t#INSPVAXA,USB3,0,47.0,FINESTEERING,2107,281659.050,02000000,471d,15824;INS_ALIGNMENT_COMPLETE,INS_RTKFIXED,37.37124867854,126.72246232189,7.9387,22.3000,-0.0180,0.2907,0.0091,-0.761412694,-0.318240084,92.179006494,0.4753,0.2827,0.5554,0.1164,0.0908,0.0769,0.1661,0.1674,5.1056,0f000001,0*0b8ce59e\n\tsystem status\tnormal 2 28.200000 0 0\trobot status\t144.136199\t124.133041\t7.938700\t-0.761413\t-0.318240\t-2.179006\t0.275000\t0.038000\n\t\n15:14:01.5\tlog_raw\tgps_raw\t\tsystem status\tnormal 2 28.100000 0 0\trobot status\t144.281252\t124.120874\t7.938900\t-0.713124\t-0.523427\t-2.080293\t0.279000\t0.033000\n\t\n15:14:02.0\tlog_raw\tgps_raw\t#INSPVAXA,USB3,0,48.0,FINESTEERING,2107,281660.050,02000000,471d,15824;INS_ALIGNMENT_COMPLETE,INS_RTKFIXED,37.37124847032,126.72246556404,7.9397,22.3000,-0.0209,0.3095,-0.0013,-0.677978130,-0.485395170,91.982371596,0.4840,0.2835,0.5609,0.1180,0.0910,0.0772,0.1661,0.1676,5.1059,0f000001,0*3e0b93c3\n\tsystem status\tnormal 2 28.100000 0 0\trobot status\t144.423383\t124.109927\t7.939700\t-0.677978\t-0.485395\t-1.982372\t0.291000\t0.029000\n\t\n15:14:02.5\tlog_raw\tgps_raw\t#INSPVAXA,USB3,0,49.0,FINESTEERING,2107,281660.550,02000000,471d,15824;INS_ALIGNMENT_COMPLETE,INS_RTKFIXED,37.37124837512,126.72246716631,7.9375,22.3000,-0.0227,0.2996,0.0028,-0.584311559,-0.386112040,91.866898679,0.4840,0.2835,0.5609,0.1180,0.0910,0.0772,0.1661,0.1676,5.1059,0f000001,0*45e2577e\n\tsystem status\tnormal 2 28.100000 0 0\trobot status\t144.565309\t124.099359\t7.937500\t-0.584312\t-0.386112\t-1.866899\t0.292000\t0.024000\n\t\n15:14:03.0\tlog_raw\tgps_raw\t#INSPVAXA,USB3,0,48.0,FINESTEERING,2107,281661.050,02000000,471d,15824;INS_ALIGNMENT_COMPLETE,INS_RTKFIXED,37.37124829104,126.72246876695,7.9348,22.3000,-0.0195,0.3013,0.0019,-0.605545922,-0.315098575,91.766604977,0.4893,0.2839,0.5649,0.1187,0.0910,0.0774,0.1661,0.1677,5.1061,0f000001,0*33d9cb01\n\tsystem status\tnormal 2 28.100000 0 0\trobot status\t144.707091\t124.090025\t7.934800\t-0.605546\t-0.315099\t-1.766605\t0.290000\t0.021000\n\t\n15:14:03.5\tlog_raw\tgps_raw\t\tsystem status\tnormal 2 28.100000 0 0\trobot status\t144.850142\t124.079476\t7.935200\t-0.604211\t-0.237981\t-1.678856\t0.302000\t0.007000\n\t\n15:14:04.0\tlog_raw\tgps_raw\t#INSPVAXA,USB3,0,48.0,FINESTEERING,2107,281662.050,02000000,471d,15824;INS_ALIGNMENT_COMPLETE,INS_RTKFIXED,37.37124811177,126.72247195093,7.9364,22.3000,-0.0115,0.2979,0.0095,-0.572003488,-0.073343292,91.548333593,0.4907,0.2839,0.5665,0.1189,0.0910,0.0775,0.1660,0.1678,5.1065,0f000001,0*28865f95\n\tsystem status\tnormal 2 28.100000 0 0\trobot status\t144.989123\t124.070124\t7.936400\t-0.572003\t-0.073343\t-1.548334\t0.295000\t0.007000\n\t\n15:14:04.5\tlog_raw\tgps_raw\t#INSPVAXA,USB3,0,49.5,FINESTEERING,2107,281662.550,02000000,471d,15824;INS_ALIGNMENT_COMPLETE,INS_RTKFIXED,37.37124803275,126.72247354020,7.9355,22.3000,-0.0061,0.2831,0.0061,-0.496782272,0.001131440,91.456585867,0.4907,0.2839,0.5665,0.1189,0.0910,0.0775,0.1660,0.1678,5.1065,0f000001,0*47f56ed7\n\tsystem status\tnormal 2 28.100000 0 0\trobot status\t145.129898\t124.061351\t7.935500\t-0.496782\t0.001131\t-1.456586\t0.276000\t0.026000\n\t\n15:14:05.0\tlog_raw\tgps_raw\t#INSPVAXA,USB3,0,49.5,FINESTEERING,2107,281663.050,02000000,471d,15824;INS_ALIGNMENT_COMPLETE,INS_RTKFIXED,37.37124795721,126.72247514952,7.9341,22.3000,-0.0032,0.2852,0.0045,-0.477077211,-0.102180757,91.467919397,0.4905,0.2838,0.5669,0.1189,0.0910,0.0775,0.1660,0.1678,5.1072,0f000001,0*7002819d\n\tsystem status\tnormal 2 28.200000 0 0\trobot status\t145.272449\t124.052965\t7.934100\t-0.477077\t-0.102181\t-1.467919\t0.272000\t0.035000\n\t\n15:14:05.5\tlog_raw\tgps_raw\t#INSPVAXA,USB3,0,50.0,FINESTEERING,2107,281663.550,02000000,471d,15824;INS_ALIGNMENT_COMPLETE,INS_RTKFIXED,37.37124785760,126.72247673495,7.9334,22.3000,-0.0075,0.2892,0.0034,-0.450270802,-0.044143313,91.482502163,0.4905,0.2838,0.5669,0.1189,0.0910,0.0775,0.1660,0.1678,5.1072,0f000001,0*8c44abc3\n\tsystem status\tnormal 2 28.200000 0 0\trobot status\t145.412884\t124.041908\t7.933400\t-0.450271\t-0.044143\t-1.482502\t0.287000\t0.016000\n\t\n15:14:06.0\tlog_raw\tgps_raw\t\tsystem status\tnormal 2 28.200000 0 0\trobot status\t145.553793\t124.030806\t7.932700\t-0.422975\t-0.035071\t-1.539826\t0.289000\t0.008000\n\t\n15:14:06.5\tlog_raw\tgps_raw\t\tsystem status\tnormal 2 28.200000 0 0\trobot status\t145.694719\t124.019126\t7.932100\t-0.556099\t-0.118368\t-1.641136\t0.294000\t-0.002000\n\t\n15:14:07.0\tlog_raw\tgps_raw\t\tsystem status\tnormal 2 28.200000 0 0\trobot status\t145.838848\t124.007271\t7.931100\t-0.699723\t-0.189031\t-1.752273\t0.297000\t-0.007000\n\t\n15:14:07.5\tlog_raw\tgps_raw\t\tsystem status\tnormal 2 28.200000 0 0\trobot status\t145.977134\t123.995521\t7.930200\t-0.725624\t-0.161796\t-1.830182\t0.296000\t-0.006000\n\t\n15:14:08.0\tlog_raw\tgps_raw\t\tsystem status\tnormal 2 28.200000 0 0\trobot status\t146.116430\t123.983395\t7.929800\t-0.705542\t-0.123551\t-1.933900\t0.298000\t-0.011000\n\t\n15:14:08.5\tlog_raw\tgps_raw\t#INSPVAXA,USB3,0,49.0,FINESTEERING,2107,281666.550,02000000,471d,15824;INS_ALIGNMENT_COMPLETE,INS_RTKFIXED,37.37124721121,126.72248621902,7.9287,22.3000,-0.0121,0.2777,0.0145,-0.831221770,-0.084392330,92.040205552,0.4814,0.2826,0.5616,0.1182,0.0910,0.0772,0.1659,0.1677,5.1107,0f000001,0*a6e58744\n\tsystem status\tnormal 2 28.200000 0 0\trobot status\t146.252967\t123.970154\t7.928700\t-0.831222\t-0.084392\t-2.040206\t0.302000\t-0.007000\n\t\n15:14:09.0\tlog_raw\tgps_raw\t#INSPVAXA,USB3,0,48.0,FINESTEERING,2107,281667.050,02000000,471d,15824;INS_ALIGNMENT_COMPLETE,INS_RTKFIXED,37.37124708689,126.72248776343,7.9278,22.3000,-0.0198,0.2843,0.0107,-0.784855196,-0.012804695,92.146893043,0.4774,0.2821,0.5586,0.1180,0.0910,0.0771,0.1659,0.1677,5.1116,0f000001,0*9d84455b\n\tsystem status\tnormal 2 28.200000 0 0\trobot status\t146.389768\t123.956354\t7.927800\t-0.784855\t-0.012805\t-2.146893\t0.303000\t-0.009000\n\t\n15:14:09.5\tlog_raw\tgps_raw\t\tsystem status\tnormal 2 28.200000 0 0\trobot status\t146.531855\t123.942035\t7.926300\t-0.788522\t-0.056258\t-2.310397\t0.297000\t-0.009000\n\t\n15:14:10.0\tlog_raw\tgps_raw\t\tsystem status\tnormal 2 28.200000 0 0\trobot status\t146.669037\t123.927984\t7.924600\t-0.772443\t-0.110200\t-2.426470\t0.297000\t-0.009000\n\t\n15:14:10.5\tlog_raw\tgps_raw\t\tsystem status\tnormal 2 28.200000 0 0\trobot status\t146.807898\t123.911429\t7.924600\t-0.795988\t-0.170149\t-2.510664\t0.300000\t-0.004000\n\t\n15:14:11.0\tlog_raw\tgps_raw\t\tsystem status\tnormal 2 28.200000 0 0\trobot status\t146.945839\t123.894882\t7.924900\t-0.749714\t-0.169943\t-2.586408\t0.300000\t-0.003000\n\t\n15:14:11.5\tlog_raw\tgps_raw\t#INSPVAXA,USB3,0,47.0,FINESTEERING,2107,281669.550,02008000,471d,15824;INS_ALIGNMENT_COMPLETE,INS_RTKFIXED,37.37124639381,126.72249565319,7.9242,22.3000,-0.0324,0.2710,-0.0043,-0.728518677,-0.210964710,92.694614055,0.4668,0.2811,0.5506,0.1171,0.0909,0.0768,0.1658,0.1676,5.1128,0f000001,0*35942a2d\n\tsystem status\tnormal 2 28.200000 0 0\trobot status\t147.088630\t123.879420\t7.924200\t-0.728519\t-0.210965\t-2.694614\t0.299000\t-0.003000\n\t\n15:14:12.0\tlog_raw\tgps_raw\t\tsystem status\tnormal 2 28.200000 0 0\trobot status\t147.228215\t123.864013\t7.922100\t-0.763620\t-0.276654\t-2.845773\t0.298000\t-0.002000\n\t\n15:14:12.5\tlog_raw\tgps_raw\t\tsystem status\tnormal 2 28.200000 0 0\trobot status\t147.367389\t123.847664\t7.919800\t-0.804800\t-0.267920\t-2.956023\t0.299000\t0.004000\n\t\n15:14:13.0\tlog_raw\tgps_raw\t#INSPVAXA,USB3,0,45.0,FINESTEERING,2107,281671.050,02008000,471d,15824;INS_ALIGNMENT_COMPLETE,INS_RTKFIXED,37.37124595365,126.72250039060,7.9180,22.3000,-0.0288,0.2756,-0.0016,-0.760823395,-0.249987892,93.080464082,0.4568,0.2803,0.5426,0.1164,0.0907,0.0766,0.1658,0.1675,5.1134,0f000001,0*bc516aa8\n\tsystem status\tnormal 2 28.200000 0 0\trobot status\t147.508263\t123.830562\t7.918000\t-0.760823\t-0.249988\t-3.080464\t0.298000\t0.000000\n\t\n15:14:13.5\tlog_raw\tgps_raw\t\tsystem status\tnormal 2 28.200000 0 0\trobot status\t147.651206\t123.814341\t7.915600\t-0.886970\t-0.340514\t-3.242034\t0.297000\t0.004000\n\t\n15:14:14.0\tlog_raw\tgps_raw\t\tsystem status\tnormal 2 28.200000 0 0\trobot status\t147.794209\t123.798366\t7.912700\t-1.083347\t-0.417187\t-3.360691\t0.302000\t0.002000\n\t\n15:14:14.5\tlog_raw\tgps_raw\t\tsystem status\tnormal 2 28.200000 0 0\trobot status\t147.932072\t123.779642\t7.909700\t-1.207404\t-0.182757\t-3.439628\t0.302000\t-0.003000\n\t\n15:14:15.0\tlog_raw\tgps_raw\t\tsystem status\tnormal 2 28.200000 0 0\trobot status\t148.076628\t123.759998\t7.906900\t-1.279448\t-0.150599\t-3.587218\t0.288000\t0.003000\n\t\n15:14:15.5\tlog_raw\tgps_raw\t\tsystem status\tnormal 2 28.200000 0 0\trobot status\t148.218981\t123.740063\t7.905500\t-1.282355\t-0.175936\t-3.644774\t0.296000\t0.001000\n\t\n15:14:16.0\tlog_raw\tgps_raw\t\tsystem status\tnormal 2 28.200000 0 0\trobot status\t148.361789\t123.719331\t7.903500\t-1.165589\t-0.117990\t-3.708978\t0.302000\t0.000000\n\t\n15:14:16.5\tlog_raw\tgps_raw\t\tsystem status\tnormal 2 28.200000 0 0\trobot status\t148.507119\t123.699632\t7.900700\t-1.250361\t-0.176704\t-3.790679\t0.295000\t0.001000\n\t\n15:14:17.0\tlog_raw\tgps_raw\t\tsystem status\tnormal 2 28.200000 0 0\trobot status\t148.651348\t123.678582\t7.899100\t-1.236438\t-0.368923\t-3.829568\t0.344000\t-0.075000\n\t\n15:14:17.5\tlog_raw\tgps_raw\t\tsystem status\tnormal 2 28.200000 0 0\trobot status\t148.798115\t123.655384\t7.896500\t-1.188609\t-0.569523\t-3.742073\t0.282000\t0.023000\n\t\n15:14:18.0\tlog_raw\tgps_raw\t\tsystem status\tnormal 2 28.100000 0 0\trobot status\t148.940214\t123.633362\t7.894900\t-1.255489\t-0.416607\t-3.558187\t0.300000\t0.017000\n\t\n15:14:18.5\tlog_raw\tgps_raw\t\tsystem status\tnormal 2 28.100000 0 0\trobot status\t149.081438\t123.612668\t7.895700\t-1.313236\t-0.235413\t-3.391774\t0.245000\t0.098000\n\t\n15:14:19.0\tlog_raw\tgps_raw\t\tsystem status\tnormal 2 28.100000 0 0\trobot status\t149.222543\t123.591760\t7.897200\t-1.300996\t-0.135698\t-3.149542\t0.295000\t0.027000\n
